vi "Experiment 15.vi"() -> ()   [LabVIEW 2026]
doc: "Experiment 15\nThis experiment is like Experiment 14 but uses while loops instead of for loops."
uses:
  <vilib>/AdvancedString/1D String Array to Delimited String (string).vi
  <vilib>/Analysis/baseanly.llb/Mean (DBL).vi
  <vilib>/Analysis/NI_AALBase.lvlib
panel:
  out "No. Of Iterations As Block Of Text (easy to copy into Excel)":string
  out "Avg. No. Of Iterations Executed - All Loops":dbl format="%.1f"
  out "No. Of Iterations Executed - Loop 2":i32
  out "Output - Loop 2":dbl[](array[numeric]) format="%.3f"
  out "No. Of Iterations Executed - Loop 1":i32
  out "Output - Loop 1":dbl[](array[numeric]) format="%.3f"
  out "Stop VI?":bool
  # "Experiment 15"
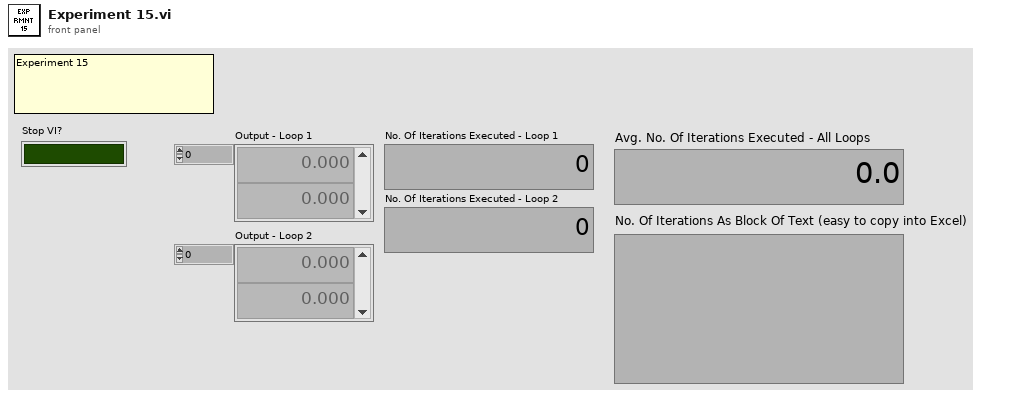
[diagram p1: front panel]
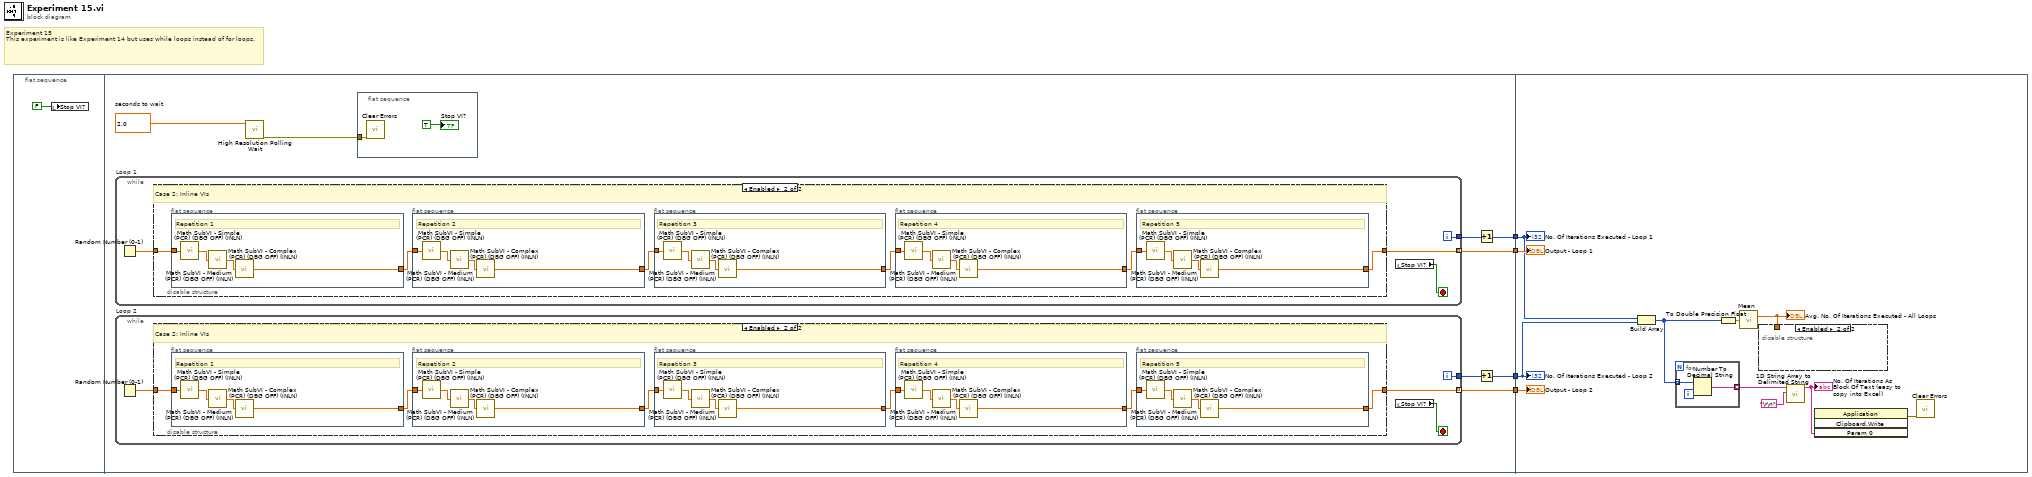
[diagram p0: block diagram]
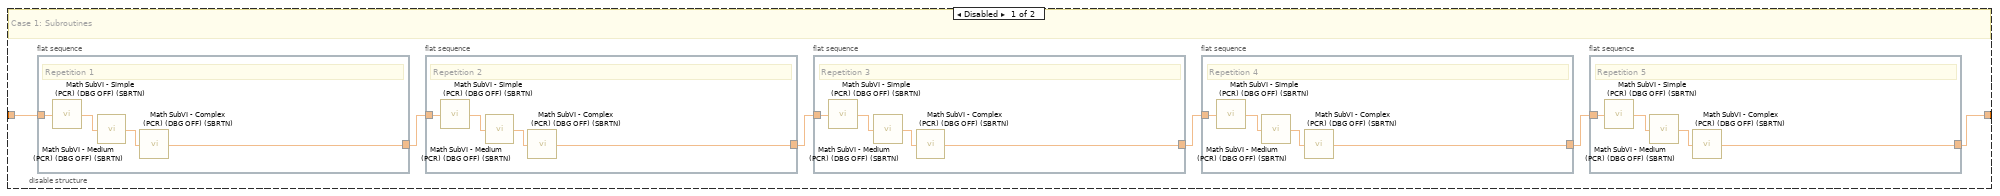
[diagram p2: hidden frame]
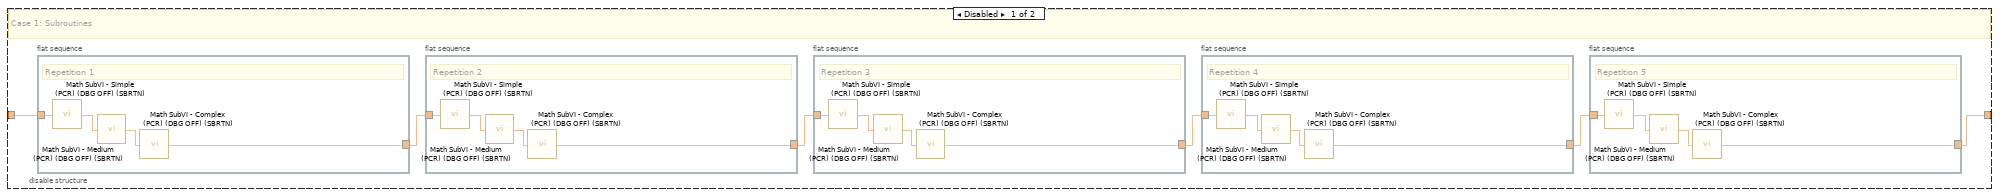
[diagram p3: hidden frame]
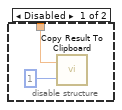
[diagram p4: hidden frame]
diagram:
  # "Experiment 15\nThis experiment is like Experiment 14 but uses while loops instead of for loops."
  n1 = flat-sequence {
    tunnel: [w11] -> w4
    tunnel: [w9] -> w3
    tunnel: [w8] -> w2
    tunnel: [w7] -> w1
    tunnel: w4 -> [w138]
    tunnel: w3 -> [w136]
    tunnel: w2 -> [w135]
    tunnel: w1 -> [w137]
    frame #0 {
      n2 = local write "Stop VI?"(FALSE) -> ()
    }
    frame #1 {
      w13 = 2.0  # seconds to wait
      n3 = while "Loop 1" {
        tunnel: [w73] -> w11 mode=indexing
        tunnel: [w74] -> w10
        i -> [w74]
        stop <- w75 stop-if-true
        n4 = Random Number (0-1)() -> (number: 0 to 1=w72:dbl)
        n5 = disable-structure shown="Enabled" {
          disable-tunnel: w72 -> [w81 w107]
          disable-tunnel: [w80 w102] -> w73
          frame Disabled {
            # "Case 1: Subroutines"
            n6 = flat-sequence {
              tunnel: w81 -> [w101]
              tunnel: [w98] -> w76
              frame #0 {
                # "Repetition 1"
                n7 = call "Math SubVI - Simple (PCR) (DBG OFF) (SBRTN).vi"("Input"=w101) -> ("Output"=w99:dbl)
                n8 = call "Math SubVI - Medium (PCR) (DBG OFF) (SBRTN).vi"("Input"=w99) -> ("Output"=w100:dbl)
                n9 = call "Math SubVI - Complex (PCR) (DBG OFF) (SBRTN).vi"("Input"=w100) -> ("Output"=w98:dbl)
              }
            }
            n10 = flat-sequence {
              tunnel: w76 -> [w97]
              tunnel: [w94] -> w79
              frame #0 {
                # "Repetition 2"
                n11 = call "Math SubVI - Simple (PCR) (DBG OFF) (SBRTN).vi"("Input"=w97) -> ("Output"=w95:dbl)
                n12 = call "Math SubVI - Medium (PCR) (DBG OFF) (SBRTN).vi"("Input"=w95) -> ("Output"=w96:dbl)
                n13 = call "Math SubVI - Complex (PCR) (DBG OFF) (SBRTN).vi"("Input"=w96) -> ("Output"=w94:dbl)
              }
            }
            n14 = flat-sequence {
              tunnel: w79 -> [w93]
              tunnel: [w90] -> w78
              frame #0 {
                # "Repetition 3"
                n15 = call "Math SubVI - Simple (PCR) (DBG OFF) (SBRTN).vi"("Input"=w93) -> ("Output"=w91:dbl)
                n16 = call "Math SubVI - Medium (PCR) (DBG OFF) (SBRTN).vi"("Input"=w91) -> ("Output"=w92:dbl)
                n17 = call "Math SubVI - Complex (PCR) (DBG OFF) (SBRTN).vi"("Input"=w92) -> ("Output"=w90:dbl)
              }
            }
            n18 = flat-sequence {
              tunnel: w78 -> [w89]
              tunnel: [w86] -> w77
              frame #0 {
                # "Repetition 4"
                n19 = call "Math SubVI - Simple (PCR) (DBG OFF) (SBRTN).vi"("Input"=w89) -> ("Output"=w87:dbl)
                n20 = call "Math SubVI - Medium (PCR) (DBG OFF) (SBRTN).vi"("Input"=w87) -> ("Output"=w88:dbl)
                n21 = call "Math SubVI - Complex (PCR) (DBG OFF) (SBRTN).vi"("Input"=w88) -> ("Output"=w86:dbl)
              }
            }
            n22 = flat-sequence {
              tunnel: w77 -> [w85]
              tunnel: [w82] -> w80
              frame #0 {
                # "Repetition 5"
                n23 = call "Math SubVI - Simple (PCR) (DBG OFF) (SBRTN).vi"("Input"=w85) -> ("Output"=w83:dbl)
                n24 = call "Math SubVI - Medium (PCR) (DBG OFF) (SBRTN).vi"("Input"=w83) -> ("Output"=w84:dbl)
                n25 = call "Math SubVI - Complex (PCR) (DBG OFF) (SBRTN).vi"("Input"=w84) -> ("Output"=w82:dbl)
              }
            }
          }
          frame Enabled {
            # "Case 2: Inline VIs"
            n26 = flat-sequence {
              tunnel: w107 -> [w127]
              tunnel: [w124] -> w106
              frame #0 {
                # "Repetition 1"
                n27 = call "Math SubVI - Simple (PCR) (DBG OFF) (INLN).vi"("Input"=w127) -> ("Output"=w125:dbl)
                n28 = call "Math SubVI - Medium (PCR) (DBG OFF) (INLN).vi"("Input"=w125) -> ("Output"=w126:dbl)
                n29 = call "Math SubVI - Complex (PCR) (DBG OFF) (INLN).vi"("Input"=w126) -> ("Output"=w124:dbl)
              }
            }
            n30 = flat-sequence {
              tunnel: w106 -> [w123]
              tunnel: [w120] -> w105
              frame #0 {
                # "Repetition 2"
                n31 = call "Math SubVI - Simple (PCR) (DBG OFF) (INLN).vi"("Input"=w123) -> ("Output"=w121:dbl)
                n32 = call "Math SubVI - Medium (PCR) (DBG OFF) (INLN).vi"("Input"=w121) -> ("Output"=w122:dbl)
                n33 = call "Math SubVI - Complex (PCR) (DBG OFF) (INLN).vi"("Input"=w122) -> ("Output"=w120:dbl)
              }
            }
            n34 = flat-sequence {
              tunnel: w105 -> [w119]
              tunnel: [w116] -> w104
              frame #0 {
                # "Repetition 3"
                n35 = call "Math SubVI - Simple (PCR) (DBG OFF) (INLN).vi"("Input"=w119) -> ("Output"=w117:dbl)
                n36 = call "Math SubVI - Medium (PCR) (DBG OFF) (INLN).vi"("Input"=w117) -> ("Output"=w118:dbl)
                n37 = call "Math SubVI - Complex (PCR) (DBG OFF) (INLN).vi"("Input"=w118) -> ("Output"=w116:dbl)
              }
            }
            n38 = flat-sequence {
              tunnel: w104 -> [w115]
              tunnel: [w112] -> w103
              frame #0 {
                # "Repetition 4"
                n39 = call "Math SubVI - Simple (PCR) (DBG OFF) (INLN).vi"("Input"=w115) -> ("Output"=w113:dbl)
                n40 = call "Math SubVI - Medium (PCR) (DBG OFF) (INLN).vi"("Input"=w113) -> ("Output"=w114:dbl)
                n41 = call "Math SubVI - Complex (PCR) (DBG OFF) (INLN).vi"("Input"=w114) -> ("Output"=w112:dbl)
              }
            }
            n42 = flat-sequence {
              tunnel: w103 -> [w111]
              tunnel: [w108] -> w102
              frame #0 {
                # "Repetition 5"
                n43 = call "Math SubVI - Simple (PCR) (DBG OFF) (INLN).vi"("Input"=w111) -> ("Output"=w109:dbl)
                n44 = call "Math SubVI - Medium (PCR) (DBG OFF) (INLN).vi"("Input"=w109) -> ("Output"=w110:dbl)
                n45 = call "Math SubVI - Complex (PCR) (DBG OFF) (INLN).vi"("Input"=w110) -> ("Output"=w108:dbl)
              }
            }
          }
        }
        n46 = local read "Stop VI?"() -> (w75:bool)
      }
      n47 = while "Loop 2" {
        tunnel: [w17] -> w7 mode=indexing
        tunnel: [w18] -> w6
        i -> [w18]
        stop <- w19 stop-if-true
        n48 = Random Number (0-1)() -> (number: 0 to 1=w16:dbl)
        n49 = disable-structure shown="Enabled" {
          disable-tunnel: w16 -> [w25 w51]
          disable-tunnel: [w24 w46] -> w17
          frame Disabled {
            # "Case 1: Subroutines"
            n50 = flat-sequence {
              tunnel: w25 -> [w45]
              tunnel: [w42] -> w20
              frame #0 {
                # "Repetition 1"
                n51 = call "Math SubVI - Simple (PCR) (DBG OFF) (SBRTN).vi"("Input"=w45) -> ("Output"=w43:dbl)
                n52 = call "Math SubVI - Medium (PCR) (DBG OFF) (SBRTN).vi"("Input"=w43) -> ("Output"=w44:dbl)
                n53 = call "Math SubVI - Complex (PCR) (DBG OFF) (SBRTN).vi"("Input"=w44) -> ("Output"=w42:dbl)
              }
            }
            n54 = flat-sequence {
              tunnel: w20 -> [w41]
              tunnel: [w38] -> w23
              frame #0 {
                # "Repetition 2"
                n55 = call "Math SubVI - Simple (PCR) (DBG OFF) (SBRTN).vi"("Input"=w41) -> ("Output"=w39:dbl)
                n56 = call "Math SubVI - Medium (PCR) (DBG OFF) (SBRTN).vi"("Input"=w39) -> ("Output"=w40:dbl)
                n57 = call "Math SubVI - Complex (PCR) (DBG OFF) (SBRTN).vi"("Input"=w40) -> ("Output"=w38:dbl)
              }
            }
            n58 = flat-sequence {
              tunnel: w23 -> [w37]
              tunnel: [w34] -> w22
              frame #0 {
                # "Repetition 3"
                n59 = call "Math SubVI - Simple (PCR) (DBG OFF) (SBRTN).vi"("Input"=w37) -> ("Output"=w35:dbl)
                n60 = call "Math SubVI - Medium (PCR) (DBG OFF) (SBRTN).vi"("Input"=w35) -> ("Output"=w36:dbl)
                n61 = call "Math SubVI - Complex (PCR) (DBG OFF) (SBRTN).vi"("Input"=w36) -> ("Output"=w34:dbl)
              }
            }
            n62 = flat-sequence {
              tunnel: w22 -> [w33]
              tunnel: [w30] -> w21
              frame #0 {
                # "Repetition 4"
                n63 = call "Math SubVI - Simple (PCR) (DBG OFF) (SBRTN).vi"("Input"=w33) -> ("Output"=w31:dbl)
                n64 = call "Math SubVI - Medium (PCR) (DBG OFF) (SBRTN).vi"("Input"=w31) -> ("Output"=w32:dbl)
                n65 = call "Math SubVI - Complex (PCR) (DBG OFF) (SBRTN).vi"("Input"=w32) -> ("Output"=w30:dbl)
              }
            }
            n66 = flat-sequence {
              tunnel: w21 -> [w29]
              tunnel: [w26] -> w24
              frame #0 {
                # "Repetition 5"
                n67 = call "Math SubVI - Simple (PCR) (DBG OFF) (SBRTN).vi"("Input"=w29) -> ("Output"=w27:dbl)
                n68 = call "Math SubVI - Medium (PCR) (DBG OFF) (SBRTN).vi"("Input"=w27) -> ("Output"=w28:dbl)
                n69 = call "Math SubVI - Complex (PCR) (DBG OFF) (SBRTN).vi"("Input"=w28) -> ("Output"=w26:dbl)
              }
            }
          }
          frame Enabled {
            # "Case 2: Inline VIs"
            n70 = flat-sequence {
              tunnel: w51 -> [w71]
              tunnel: [w68] -> w50
              frame #0 {
                # "Repetition 1"
                n71 = call "Math SubVI - Simple (PCR) (DBG OFF) (INLN).vi"("Input"=w71) -> ("Output"=w69:dbl)
                n72 = call "Math SubVI - Medium (PCR) (DBG OFF) (INLN).vi"("Input"=w69) -> ("Output"=w70:dbl)
                n73 = call "Math SubVI - Complex (PCR) (DBG OFF) (INLN).vi"("Input"=w70) -> ("Output"=w68:dbl)
              }
            }
            n74 = flat-sequence {
              tunnel: w50 -> [w67]
              tunnel: [w64] -> w49
              frame #0 {
                # "Repetition 2"
                n75 = call "Math SubVI - Simple (PCR) (DBG OFF) (INLN).vi"("Input"=w67) -> ("Output"=w65:dbl)
                n76 = call "Math SubVI - Medium (PCR) (DBG OFF) (INLN).vi"("Input"=w65) -> ("Output"=w66:dbl)
                n77 = call "Math SubVI - Complex (PCR) (DBG OFF) (INLN).vi"("Input"=w66) -> ("Output"=w64:dbl)
              }
            }
            n78 = flat-sequence {
              tunnel: w49 -> [w63]
              tunnel: [w60] -> w48
              frame #0 {
                # "Repetition 3"
                n79 = call "Math SubVI - Simple (PCR) (DBG OFF) (INLN).vi"("Input"=w63) -> ("Output"=w61:dbl)
                n80 = call "Math SubVI - Medium (PCR) (DBG OFF) (INLN).vi"("Input"=w61) -> ("Output"=w62:dbl)
                n81 = call "Math SubVI - Complex (PCR) (DBG OFF) (INLN).vi"("Input"=w62) -> ("Output"=w60:dbl)
              }
            }
            n82 = flat-sequence {
              tunnel: w48 -> [w59]
              tunnel: [w56] -> w47
              frame #0 {
                # "Repetition 4"
                n83 = call "Math SubVI - Simple (PCR) (DBG OFF) (INLN).vi"("Input"=w59) -> ("Output"=w57:dbl)
                n84 = call "Math SubVI - Medium (PCR) (DBG OFF) (INLN).vi"("Input"=w57) -> ("Output"=w58:dbl)
                n85 = call "Math SubVI - Complex (PCR) (DBG OFF) (INLN).vi"("Input"=w58) -> ("Output"=w56:dbl)
              }
            }
            n86 = flat-sequence {
              tunnel: w47 -> [w55]
              tunnel: [w52] -> w46
              frame #0 {
                # "Repetition 5"
                n87 = call "Math SubVI - Simple (PCR) (DBG OFF) (INLN).vi"("Input"=w55) -> ("Output"=w53:dbl)
                n88 = call "Math SubVI - Medium (PCR) (DBG OFF) (INLN).vi"("Input"=w53) -> ("Output"=w54:dbl)
                n89 = call "Math SubVI - Complex (PCR) (DBG OFF) (INLN).vi"("Input"=w54) -> ("Output"=w52:dbl)
              }
            }
          }
        }
        n90 = local read "Stop VI?"() -> (w19:bool)
      }
      n91 = call <vilib>:"High Resolution Polling Wait.vi"("seconds to wait"=w13) -> ("error out"=w12:errorcluster)  [unwired: 10 in]
      n92 = flat-sequence {
        tunnel: w12 -> [w14]
        frame #0 {
          n93 = call <vilib>:"Clear Errors.vi"("error in (no error)"=w14) -> ()  [unwired: 5 in, 2 out]
          "Stop VI?" <- TRUE
        }
      }
      n94 = Increment(x=w10) -> (x+1=w9:i32)
      n95 = Increment(x=w6) -> (x+1=w8:i32)
    }
    frame #2 {
      n96 = Build Array(w136, w135) -> (w132:i32[])
      n97 = for {
        tunnel: w132 -> [w142] mode=indexing
        tunnel: [w141] -> w131 mode=indexing
        n98 = Number To Decimal String(number=w142) -> (decimal integer string=w141:string)  [unwired: 1 in]
      }
      n99 = To Double Precision Float(number=w132) -> (double precision float=w133:dbl[])
      n100 = call-poly <vilib>:"Mean.vi"("X"=w133) -> ("mean"=w134:dbl)  [unwired: 1 out]
      "Avg. No. Of Iterations Executed - All Loops" <- w134
      n101 = disable-structure shown="Enabled" {
        disable-tunnel: w134 -> [w140 _]
        frame Disabled {
          n102 = call "Copy Result To Clipboard.vi"("No. Of Decimal Places (6)"=u32 1, "Input"=w140) -> ()
        }
        frame Enabled {
        }
      }
      n103 = call-poly <vilib>:"1D String Array to Delimited String.vi"("delimiter"="\r\n", "string array"=w131) -> ("delimited string"=w128:string)  [unwired: 9 in]
      "No. Of Iterations As Block Of Text (easy to copy into Excel)" <- w128
      n104 = invoke class="Application" method="Clipboard.Write"("Param 0"=w128) -> (error out=w129:errorcluster)  [unwired: 3 in, 3 out]
      n105 = call <vilib>:"Clear Errors.vi"("error in (no error)"=w129) -> ()  [unwired: 5 in, 2 out]
      "No. Of Iterations Executed - Loop 1" <- w136
      "Output - Loop 1" <- w138
      "No. Of Iterations Executed - Loop 2" <- w135
      "Output - Loop 2" <- w137
    }
  }
